vi "Get Type.vi"(8 "error in (no error)":errorcluster, 11 "Item in":refnum<class "Item.lvclass">) -> (0 "error out":errorcluster, 2 "Item Type":T1, 3 "Item out":refnum<class "Item.lvclass">)   [LabVIEW 2020, in "Item.lvclass"]
uses:
  Item.lvclass
  Item Type.ctl
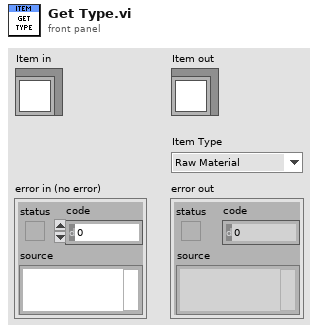
[diagram p1: front panel]
types:
  T1 = typedef "Item.lvclass/Item Type.ctl" = enum16{"Raw Material", "Component", "Module", "Product"}
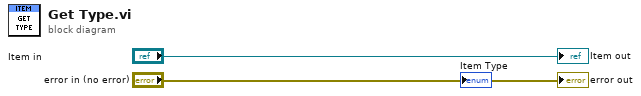
[diagram p0: block diagram]
diagram:
  "error out" <- "error in (no error)"
  "Item out" <- "Item in"
